vi "Send Message.vi"(8 "Error In":errorcluster, 10 "IMessage":refnum<class "IMessage.lvclass">, 11 "Communicator in":refnum<class "Communicator.lvclass">) -> (0 "Error Out":errorcluster, 3 "Communicator out":refnum<class "Communicator.lvclass">)   [LabVIEW 2025, in "Communicator.lvclass"]
uses:
  Communicator.lvclass
  Interfaces/IMessage/IMessage.lvclass
  Interfaces/ICommunicate/ICommunicate.lvclass
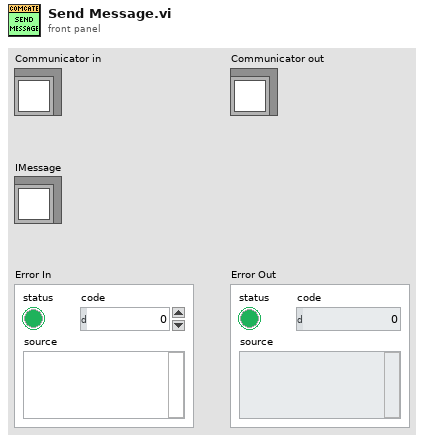
[diagram p1: front panel]
types:
  T1 = typedef "Communicator.lvclass/ObjectAttributes.ctl" = cluster{"IConfigure":refnum<class "IConfigure.lvclass">, "Worker Enqueuer":refnum<class "Message Enqueuer.lvclass">, "Start Counter":i32, "Msg Sent":refnum<user-event>}
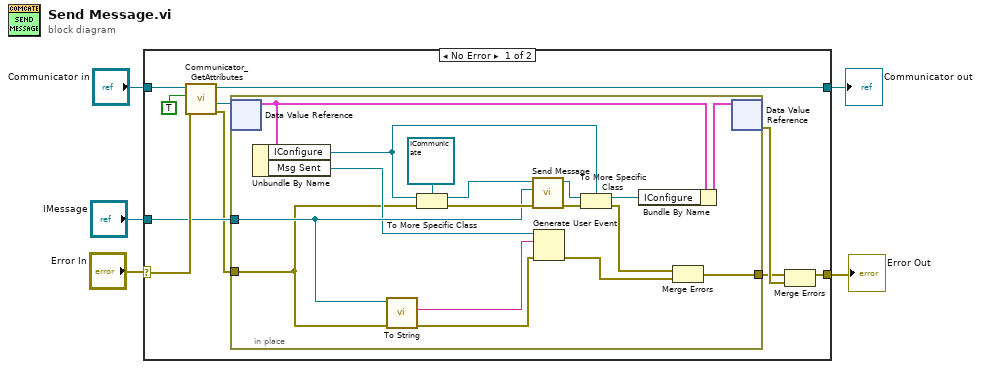
[diagram p0: block diagram]
diagram:
  n1 = case shown="No Error" "Error In" {
    selector: "Error In" -> [w14 w34]
    tunnel: [w12 w34] -> w4
    tunnel: [w13 w33] -> w2
    tunnel: "Communicator in" -> [w15 w33]
    tunnel: "IMessage" -> [w9 _]
    frame No Error {
      n2 = call "Communicator_GetAttributes.vi"("Error In"=w14, "OnlyGetDvrReference(False)"=TRUE, "Communicator in"=w15) -> ("Error Out"=w8:errorcluster, "DataRef"=w11:refnum<data-value>, "Communicator out"=w13:refnum<class "Communicator.lvclass">)  [unwired: 5 in, 1 out]
      n3 = in-place {
        in-place-border: w9 -> [w22]
        in-place-border: [w20] -> w6
        in-place-border: w8 -> [w17]
        n4 = in-place-dvr #1(w11) -> (w31:T1)  [unwired: 1 out]
        n5 = Unbundle By Name(w31) -> ("IConfigure"=w27:refnum<class "IConfigure.lvclass">, "Msg Sent"=w18:refnum<user-event>)
        n6 = call-dynamic "To String.vi"("error in"=w17, "IMessage in"=w22) -> ("error out"=w21:errorcluster, "Stringified"=w16:string)  [unwired: 7 in, 1 out]
        n7 = To More Specific Class(target class=refnum<class "ICommunicate.lvclass"> refnum ("ICommunicate.lvclass"), reference=w27, error in=w17) -> (specific class reference=w25:refnum<class "ICommunicate.lvclass">, error out=w23:errorcluster)
        n8 = call-dynamic "Send Message.vi"("error in"=w23, "IMessage"=w22, "ICommunicate in"=w25) -> ("error out"=w24:errorcluster, "ICommunicate out"=w29:refnum<class "ICommunicate.lvclass">)  [unwired: 7 in]
        n9 = Generate User Event(user event=w18, event data cluster=w16, error in=w21) -> (error out=w19:errorcluster)  [unwired: 1 in, 1 out]
        n10 = To More Specific Class(target class=w27, reference=w29, error in=w24) -> (specific class reference=w28:refnum<class "IConfigure.lvclass">, error out=w26:errorcluster)
        n11 = Bundle By Name(cluster=w31, "IConfigure"=w28) -> (w32:T1)
        n12 = Merge Errors(w26, w19) -> (w20:errorcluster)
        n13 = in-place-dvr #1(w32) -> (w7:errorcluster)  [unwired: 1 out]
      }
      n14 = Merge Errors(w6, w7) -> (w12:errorcluster)
    }
    frame Error {
    }
  }
  "Error Out" <- w4
  "Communicator out" <- w2
